vi "CalculateIndex.vi"(2 "First Frm Indx":dbl, 3 "Cam Frst Frm":dbl, 4 "# of Vessels":dbl, 5 "Frm #":dbl) -> (0 "Vessel #":dbl, 1 "Frm Indx":dbl)   [LabVIEW 2012]
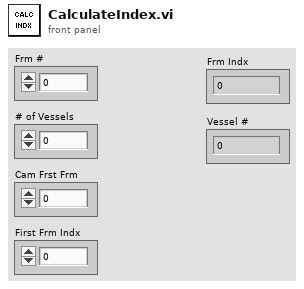
[diagram p1: front panel]
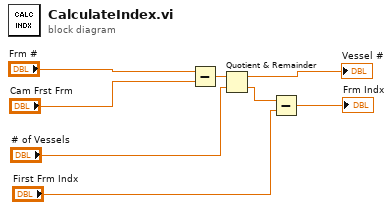
[diagram p0: block diagram]
diagram:
  n1 = Subtract(x="Frm #", y="Cam Frst Frm") -> (x-y=w8:dbl)
  n2 = Quotient & Remainder(x=w8, y="# of Vessels") -> (x-y*floor(x/y)=→"Vessel #":dbl, floor(x/y)=w7:dbl)
  n3 = Subtract(x=w7, y="First Frm Indx") -> (x-y=→"Frm Indx":dbl)
